vi "Flatten to YAML.vi"(4 "Condensed?":bool, 6 "No Label?":bool, 8 "error in (no error)":errorcluster, 11 "Anything":variant) -> (0 "error out":errorcluster, 3 "YAML String":string)   [LabVIEW 2015, in "YAML Parser.lvlib"]
uses:
  YAML Parser.lvlib
  <vilib>/Utility/Data Type/NI_Data Type.lvlib
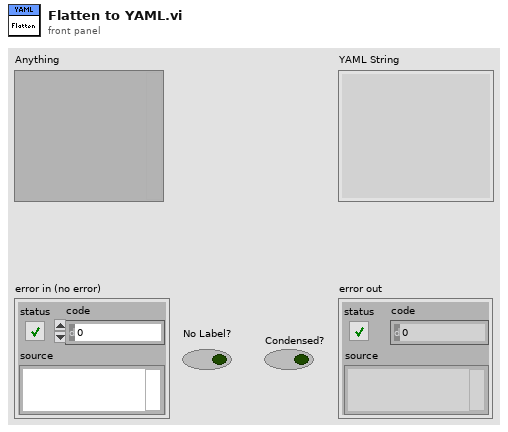
[diagram p1: front panel]
types:
  T1 = typedef "NI_Data Type.lvlib/Data Type.ctl" = enum8{"Invalid Type", "Void", "I8", "I16", "I32", "I64", "U8", "U16", "U32", "U64", "Single Float", "Double Float", "Extended Float", "Single Complex", "Double Complex", "Extended Complex", "Enum U8", "Enum U16", "Enum U32", "Enum U64", "Single Float With Unit", "Double Float With Unit", "Extended Float With Unit", "Single Complex with Unit", "Double Complex with Unit", "Extended Complex with Unit", "Boolean", "String", "Path", "Picture", "Tag", "Array", "Cluster", "Variant", "LV Variant", "Waveform", "Timestamp", "Digital Waveform", "Digital Data", "ExpressData", "Refnum", "External Data", "VI", "Poly VI", "LabVIEW Class Instance", "Fixed Point"}
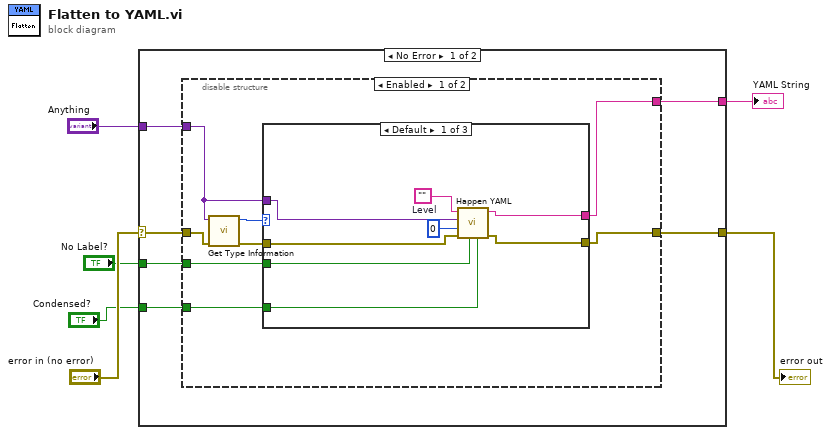
[diagram p0: block diagram]
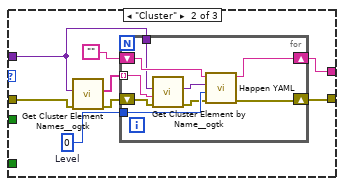
[diagram p2: hidden frame]
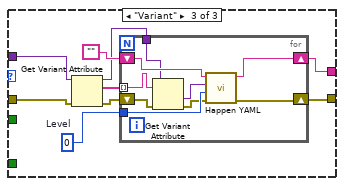
[diagram p3: hidden frame]
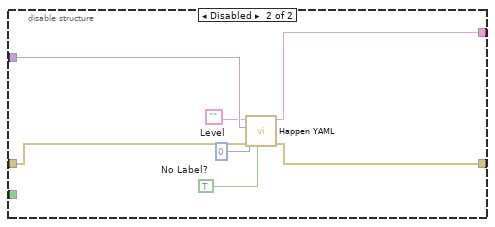
[diagram p4: hidden frame]
diagram:
  n1 = case shown="No Error" "error in (no error)" {
    selector: "error in (no error)" -> [w12 w71]
    tunnel: [w11 w71] -> w5
    tunnel: "Anything" -> [w10 _]
    tunnel: [w9 _] -> w3
    tunnel: "No Label?" -> [w8 _]
    tunnel: "Condensed?" -> [w7 _]
    frame No Error {
      n2 = disable-structure shown="Enabled" {
        disable-tunnel: w12 -> [w18 w70]
        disable-tunnel: [w17 w69] -> w11
        disable-tunnel: w10 -> [w16 w68]
        disable-tunnel: [w15 w64] -> w9
        disable-tunnel: w8 -> [w14 _]
        disable-tunnel: w7 -> [w13 _]
        frame Enabled {
          n3 = call <vilib>:"Get Type Information.vi"("error in (no error)"=w18, "Variant"=w16) -> ("error out"=w19:errorcluster, "Type"=w20:T1)  [unwired: 5 in, 3 out]
          n4 = case shown="Default" w20 {
            tunnel: w19 -> [w26 w32 w50]
            tunnel: w16 -> [w24 w29 w49]
            tunnel: [w25 w36 w54] -> w17
            tunnel: [w23 w35 w53] -> w15
            tunnel: w14 -> [w22 _ _]
            tunnel: w13 -> [w21 _ _]
            frame Default {
              w27 = u32 0  # Level
              n5 = call "Happen YAML.vi"("Condensed?"=w21, "No Label?"=w22, "error in (no error)"=w26, "Level"=w27, "Anything"=w24, "YAML String in"="") -> ("error out"=w25:errorcluster, "YAML String out"=w23:string)  [unwired: 4 in]
            }
            frame "Cluster" {
              w33 = u32 0  # Level
              n6 = call <userlib>:"Get Cluster Element Names__ogtk.vi"("error in (no error)"=w32, "Cluster"=w29) -> ("error out"=w31:errorcluster, "Element Names"=w30:string[])  [unwired: 8 in]
              n7 = for {
                tunnel: w30 -> [w38] mode=indexing
                shift-right: [w45] -> w36
                shift-left: w31 -> [w41]
                shift-right: [w42] -> w35
                shift-left: "" -> [w43]
                tunnel: w33 -> [w44]
                tunnel: w29 -> [w39]
                n8 = call <userlib>:"Get Cluster Element by Name__ogtk.vi"("error in (no error)"=w41, "Element Name"=w38, "Cluster"=w39) -> ("error out"=w40:errorcluster, "VElement"=w37:variant)  [unwired: 6 in, 1 out]
                n9 = call "Happen YAML.vi"("error in (no error)"=w40, "Level"=w44, "Anything"=w37, "YAML String in"=w43) -> ("error out"=w45:errorcluster, "YAML String out"=w42:string)  [unwired: 6 in]
              }
            }
            frame "Variant" {
              w51 = u32 0  # Level
              n10 = Get Variant Attribute(Variant=w49, error in=w50) -> (duplicate Variant=w48:variant, names=w46:string[], error out=w47:errorcluster)  [unwired: 2 in, 1 out]
              n11 = for {
                shift-right: [w63] -> w54
                shift-left: w47 -> [w59]
                shift-right: [w60] -> w53
                shift-left: "" -> [w61]
                tunnel: w51 -> [w62]
                tunnel: w48 -> [w56]
                tunnel: w46 -> [w57] mode=indexing
                n12 = Get Variant Attribute(Variant=w56, name=w57, error in=w59) -> (value=w55:variant, error out=w58:errorcluster)  [unwired: 1 in, 2 out]
                n13 = call "Happen YAML.vi"("error in (no error)"=w58, "Level"=w62, "Anything"=w55, "YAML String in"=w61) -> ("error out"=w63:errorcluster, "YAML String out"=w60:string)  [unwired: 6 in]
              }
            }
          }
        }
        frame Disabled {
          w65 = TRUE  # No Label?
          w66 = u32 0  # Level
          n14 = call "Happen YAML.vi"("No Label?"=w65, "error in (no error)"=w70, "Level"=w66, "Anything"=w68, "YAML String in"="") -> ("error out"=w69:errorcluster, "YAML String out"=w64:string)  [unwired: 5 in]
        }
      }
    }
    frame Error {
    }
  }
  "error out" <- w5
  "YAML String" <- w3
